vi "SetViews.vi"(8 "error in (no error)":errorcluster, 10 "Data":T1(array[cluster]), 11 "ViewMgr in":refnum<class "ViewMgr.lvclass">) -> (0 "error out":errorcluster, 3 "ViewMgr out":refnum<class "ViewMgr.lvclass">)   [LabVIEW 2020, in "CSM-TagDBDisplayContainer.lvlib" / "ViewMgr.lvclass"]
uses:
  ViewMgr.lvclass
  ViewMgr.lvclass/ViewMgr.ctl
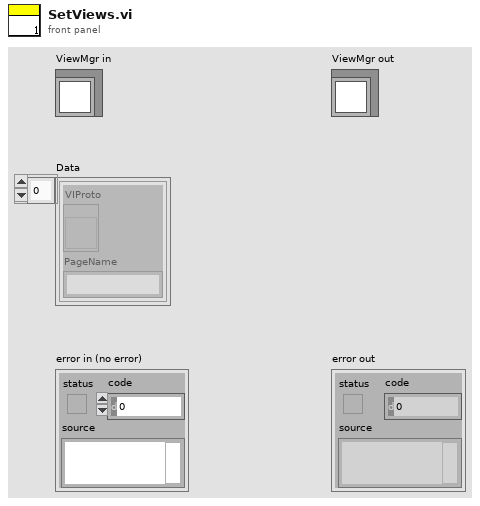
[diagram p1: front panel]
types:
  T1 = cluster{"VIProto":refnum<vi>, "PageName":string}[]
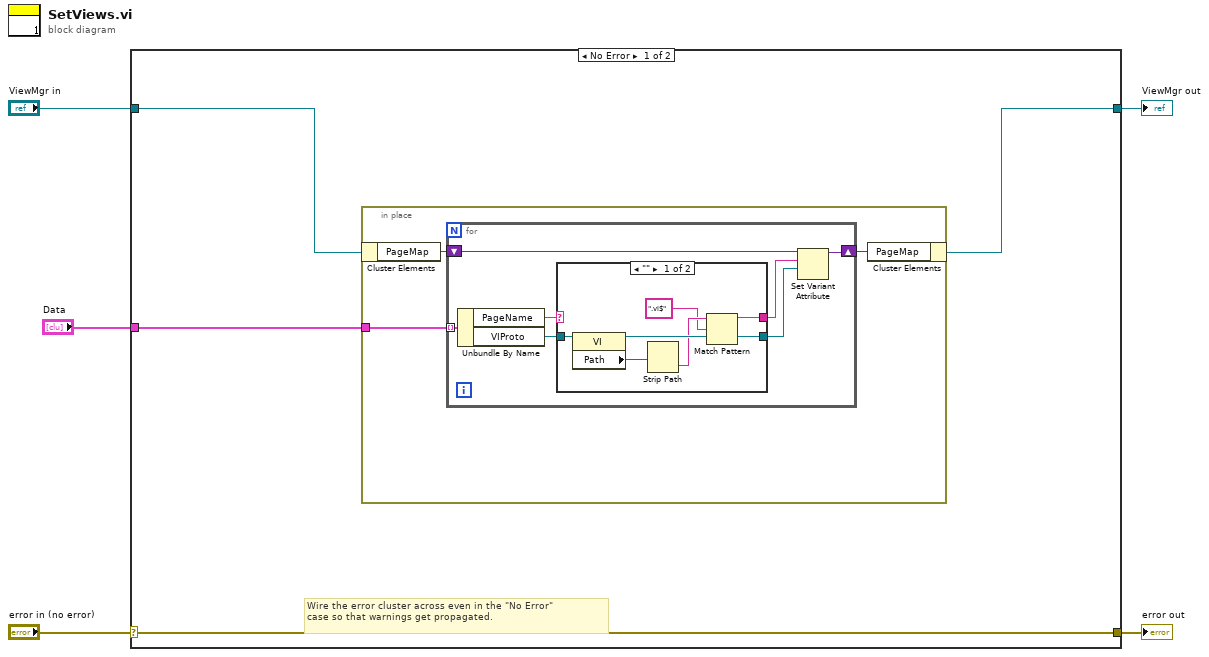
[diagram p0: block diagram]
diagram:
  n1 = case shown="No Error" "error in (no error)" {
    selector: "error in (no error)" -> [w9 w29]
    tunnel: [w9 w29] -> w4
    tunnel: [w7 w28] -> w2
    tunnel: "ViewMgr in" -> [w8 w28]
    tunnel: "Data" -> [w6 _]
    frame No Error {
      # "Wire the error cluster across even in the \"No Error\"\ncase so that warnings get propagated."
      n2 = in-place {
        in-place-border: w6 -> [w10]
        n3 = in-place-cluster #1(w8) -> ("PageMap"=w12:variant)
        n4 = for {
          shift-right: [w18] -> w11
          shift-left: w12 -> [w19]
          tunnel: w10 -> [w17] mode=indexing
          n5 = Unbundle By Name(w17) -> ("PageName"=w16:string, "VIProto"=w14:refnum<vi>)
          n6 = case shown="\"\"" w16 {
            selector: w16 -> [_ w26]
            tunnel: [w24 w27] -> w15
            tunnel: w14 -> [w25 w27]
            tunnel: [w21 w26] -> w13
            frame "" {
              n7 = property class="VI"(reference=w25) -> (reference out=w24:refnum<vi>, "Path"=w23:path)  [unwired: 1 in, 1 out]
              n8 = Strip Path(path=w23) -> (name=w22:string)  [unwired: 1 out]
              n9 = Match Pattern(string=w22, regular expression=".vi$" ("string")) -> (before substring=w21:string)  [unwired: 1 in, 3 out]
            }
            frame Default {
            }
          }
          n10 = Set Variant Attribute(Variant=w19, name=w13, value=w15) -> (Variant out=w18:variant)  [unwired: 1 in, 2 out]
        }
        n11 = in-place-cluster #1("PageMap"=w11) -> (w7:refnum<class "ViewMgr.lvclass">)
      }
    }
    frame Error {
    }
  }
  "error out" <- w4
  "ViewMgr out" <- w2
